vi "Telescope Stop.vi"(8 "error in (no error)":errorcluster, 11 "Telescope Simulator in":refnum<class "Telescope Simulator.lvclass">) -> (0 "error out":errorcluster, 3 "Telescope Simulator out":refnum<class "Telescope Simulator.lvclass">)   [LabVIEW 2024, in "Telescope Simulator.lvclass"]
uses:
  Telescope Simulator.lvclass
  Telescope enum Status.ctl
  Telescope Simulator.lvclass/Telescope Simulator.ctl
  Telescope.lvclass
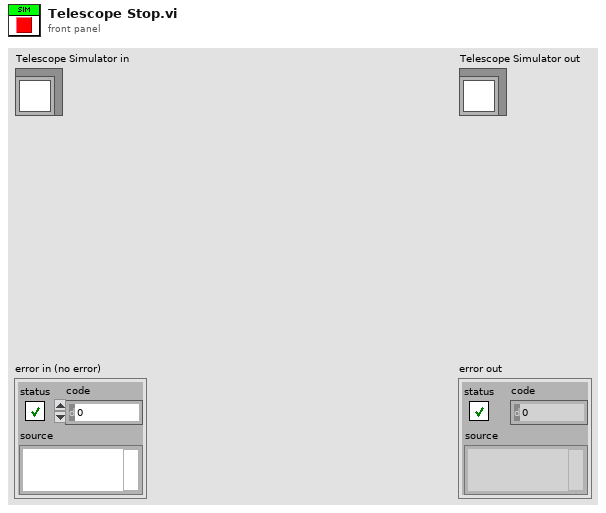
[diagram p1: front panel]
types:
  T1 = typedef "Telescope.lvclass/Telescope enum Status.ctl" = enum16{"Initializing", "Ready", "Moving", "Focusing", "Error"}
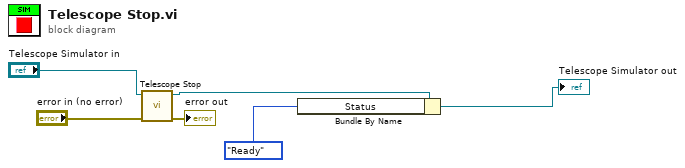
[diagram p0: block diagram]
diagram:
  n1 = call-parent "Telescope Stop.vi"("error in (no error)"="error in (no error)", "Telescope in"="Telescope Simulator in") -> ("error out"=→"error out":errorcluster, "Telescope out"=w3:refnum<class "Telescope Simulator.lvclass">)  [unwired: 8 in]
  n2 = Bundle By Name(cluster=w3, "Status"=Telescope_enum_Status."Ready" ("Telescope Status.Status")) -> (→"Telescope Simulator out":refnum<class "Telescope Simulator.lvclass">)
